vi "Untitled 1.vi"() -> ()   [LabVIEW 2015]
uses:
  Windows/System32/user32.dll
panel:
  out "Binary Netmask":string
  out "String 2":string
  out "Hosts":string
  out "Host max":string
  out "Host min":string
  out "Broadcast":string
  out "Network":string
  out "Wildcard":string
  out "Netmask":string
  out "Address":string
  in  "INFO":T1
  # "."
  # "."
  # "."
  # "(i.e /24)"
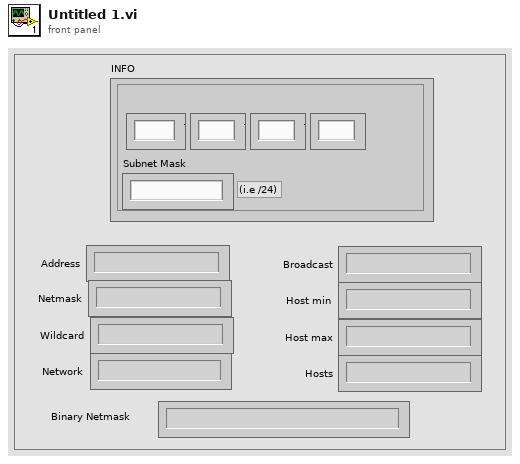
[diagram p1: front panel]
types:
  T1 = cluster{"Subnet Mask":string, "0":string, "1":string, "2":string, "3":string}
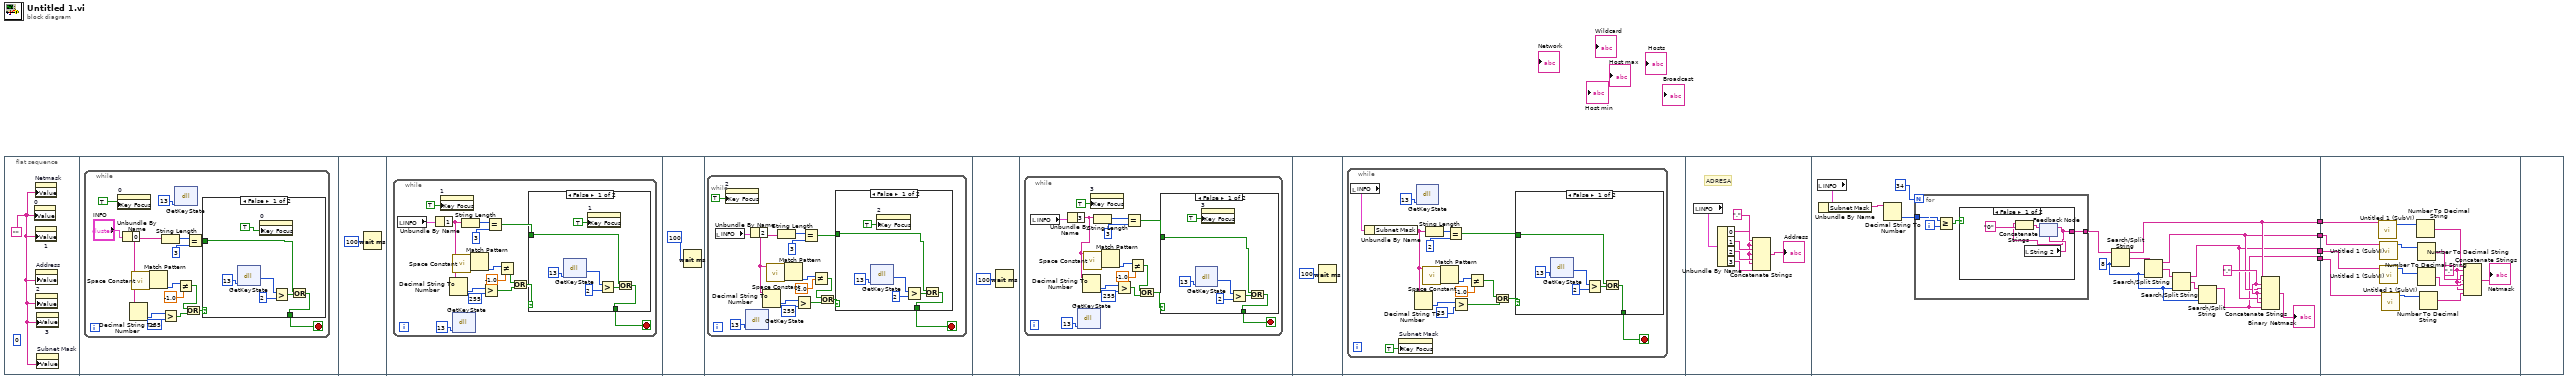
[diagram p0: block diagram]
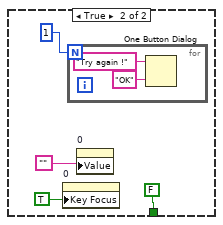
[diagram p2: hidden frame]
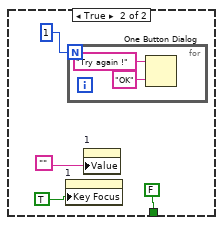
[diagram p3: hidden frame]
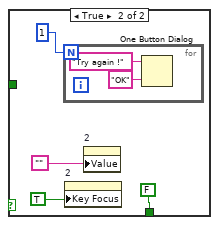
[diagram p4: hidden frame]
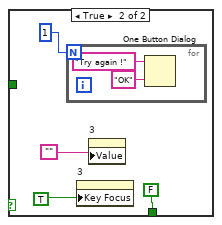
[diagram p5: hidden frame]
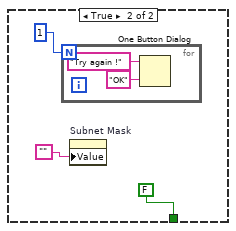
[diagram p6: hidden frame]
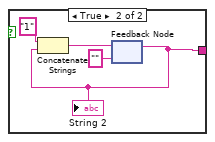
[diagram p7: hidden frame]
diagram:
  n1 = flat-sequence {
    tunnel: [w163] -> w4
    tunnel: [w162] -> w3
    tunnel: [w161] -> w2
    tunnel: [w160] -> w1
    tunnel: w4 -> [w200]
    tunnel: w3 -> [w198]
    tunnel: w2 -> [w197]
    tunnel: w1 -> [w196]
    frame #0 {
      (unwired) 0 ("return type")
      w5 = ""
      n2 = property on="0" class="Str"("Value"=w5) -> ()  [unwired: 2 in, 2 out]
      n3 = property on="Netmask" class="Str"("Value"=w5) -> ()  [unwired: 2 in, 2 out]
      n4 = property on="1" class="Str"("Value"=w5) -> ()  [unwired: 2 in, 2 out]
      n5 = property on="Address" class="Str"("Value"=w5) -> ()  [unwired: 2 in, 2 out]
      n6 = property on="2" class="Str"("Value"=w5) -> ()  [unwired: 2 in, 2 out]
      n7 = property on="3" class="Str"("Value"=w5) -> ()  [unwired: 2 in, 2 out]
      n8 = property on="Subnet Mask" class="Str"("Value"=w5) -> ()  [unwired: 2 in, 2 out]
    }
    frame #1 {
      n9 = while {
        stop <- w15 stop-if-true
        n10 = property on="0" class="Str"("Key Focus"=TRUE) -> ()  [unwired: 2 in, 2 out]
        n11 = Unbundle By Name("INFO") -> ("0"=w11:string)
        n12 = Decimal String To Number(string=w11) -> (number=w17:i32)  [unwired: 2 in, 1 out]
        n13 = call <vilib>:"Space Constant.vi"() -> ("String"=w13:string)
        n14 = Match Pattern(string=w11, regular expression=w13) -> (offset past match=w12:i32)  [unwired: 1 in, 3 out]
        n15 = String Length(string=w11) -> (length=w19:i32)
        n16 = Greater?(x=w17, y=255) -> (0:w9:bool)
        n17 = dll-call lib="C:/Windows/System32/user32.dll" fn="GetKeyState"("vkey"=13) -> ()  [unwired: 5 in, 2 out]
        n18 = Not Equal?(x=w12, y=-1.0) -> (x != y?=w8:bool)
        n19 = Or(x=w8, y=w9) -> (x .or. y?=w7:bool)
        n20 = Equal?(x=w19, y=3) -> (x = y?=w14:bool)
        n21 = case shown="False" w7 {
          tunnel: [w22 FALSE] -> w15
          tunnel: w14 -> [w23 _]
          frame False {
            n22 = dll-call lib="C:/Windows/System32/user32.dll" fn="GetKeyState"("vkey"=13) -> ("return type"=w26:i32)  [unwired: 4 in, 2 out]
            n23 = property on="0" class="Str"("Key Focus"=TRUE) -> ()  [unwired: 2 in, 2 out]
            n24 = Greater?(x=w26, y=2) -> (0:w24:bool)
            n25 = Or(x=w23, y=w24) -> (x .or. y?=w22:bool)
          }
          frame True {
            n26 = property on="0" class="Str"("Key Focus"=TRUE) -> ()  [unwired: 2 in, 2 out]
            n27 = for {
              N: 1 -> [_]
              n28 = One Button Dialog(message="Try again !", button name ("OK")="OK") -> ()  [unwired: 1 out]
            }
            n29 = property on="0" class="Str"("Value"="") -> ()  [unwired: 2 in, 2 out]
          }
        }
      }
    }
    frame #2 {
      n30 = Wait (ms)(milliseconds to wait=u32 100) -> ()  [unwired: 1 out]
    }
    frame #3 {
      n31 = while {
        stop <- w44 stop-if-true
        n32 = local read "INFO"() -> (w51:T1)
        n33 = Unbundle By Name(w51) -> ("1"=w41:string)
        n34 = property on="1" class="Str"("Key Focus"=TRUE) -> ()  [unwired: 2 in, 2 out]
        n35 = Decimal String To Number(string=w41) -> (number=w47:i32)  [unwired: 2 in, 1 out]
        n36 = dll-call lib="C:/Windows/System32/user32.dll" fn="GetKeyState"("vkey"=13) -> ()  [unwired: 5 in, 2 out]
        n37 = call <vilib>:"Space Constant.vi"() -> ("String"=w43:string)
        n38 = String Length(string=w41) -> (length=w50:i32)
        n39 = Match Pattern(string=w41, regular expression=w43) -> (offset past match=w42:i32)  [unwired: 1 in, 3 out]
        n40 = Greater?(x=w47, y=255) -> (0:w39:bool)
        n41 = Equal?(x=w50, y=3) -> (x = y?=w45:bool)
        n42 = Not Equal?(x=w42, y=-1.0) -> (x != y?=w38:bool)
        n43 = Or(x=w38, y=w39) -> (x .or. y?=w40:bool)
        n44 = case shown="False" w40 {
          tunnel: [w52 FALSE] -> w44
          tunnel: w45 -> [w53 _]
          frame False {
            n45 = dll-call lib="C:/Windows/System32/user32.dll" fn="GetKeyState"("vkey"=13) -> ("return type"=w56:i32)  [unwired: 4 in, 2 out]
            n46 = property on="1" class="Str"("Key Focus"=TRUE) -> ()  [unwired: 2 in, 2 out]
            n47 = Greater?(x=w56, y=2) -> (0:w54:bool)
            n48 = Or(x=w53, y=w54) -> (x .or. y?=w52:bool)
          }
          frame True {
            n49 = property on="1" class="Str"("Key Focus"=TRUE) -> ()  [unwired: 2 in, 2 out]
            n50 = for {
              N: 1 -> [_]
              n51 = One Button Dialog(message="Try again !", button name ("OK")="OK") -> ()  [unwired: 1 out]
            }
            n52 = property on="1" class="Str"("Value"="") -> ()  [unwired: 2 in, 2 out]
          }
        }
      }
    }
    frame #4 {
      n53 = Wait (ms)(milliseconds to wait=u32 100) -> ()  [unwired: 1 out]
    }
    frame #5 {
      n54 = while {
        stop <- w74 stop-if-true
        n55 = local read "INFO"() -> (w79:T1)
        n56 = property on="2" class="Str"("Key Focus"=TRUE) -> ()  [unwired: 2 in, 2 out]
        n57 = dll-call lib="C:/Windows/System32/user32.dll" fn="GetKeyState"("vkey"=13) -> ()  [unwired: 5 in, 2 out]
        n58 = Unbundle By Name(w79) -> ("2"=w68:string)
        n59 = Decimal String To Number(string=w68) -> (number=w77:i32)  [unwired: 2 in, 1 out]
        n60 = call <vilib>:"Space Constant.vi"() -> ("String"=w73:string)
        n61 = String Length(string=w68) -> (length=w81:i32)
        n62 = Match Pattern(string=w68, regular expression=w73) -> (offset past match=w72:i32)  [unwired: 1 in, 3 out]
        n63 = Greater?(x=w77, y=255) -> (0:w69:bool)
        n64 = Equal?(x=w81, y=3) -> (x = y?=w75:bool)
        n65 = Not Equal?(x=w72, y=-1.0) -> (x != y?=w70:bool)
        n66 = Or(x=w70, y=w69) -> (x .or. y?=w71:bool)
        n67 = case shown="False" w71 {
          tunnel: [w82 FALSE] -> w74
          tunnel: w75 -> [w83 _]
          frame False {
            n68 = dll-call lib="C:/Windows/System32/user32.dll" fn="GetKeyState"("vkey"=13) -> ("return type"=w86:i32)  [unwired: 4 in, 2 out]
            n69 = property on="2" class="Str"("Key Focus"=TRUE) -> ()  [unwired: 2 in, 2 out]
            n70 = Greater?(x=w86, y=2) -> (0:w84:bool)
            n71 = Or(x=w83, y=w84) -> (x .or. y?=w82:bool)
          }
          frame True {
            n72 = for {
              N: 1 -> [_]
              n73 = One Button Dialog(message="Try again !", button name ("OK")="OK") -> ()  [unwired: 1 out]
            }
            n74 = property on="2" class="Str"("Key Focus"=TRUE) -> ()  [unwired: 2 in, 2 out]
            n75 = property on="2" class="Str"("Value"="") -> ()  [unwired: 2 in, 2 out]
          }
        }
      }
    }
    frame #6 {
      n76 = Wait (ms)(milliseconds to wait=u32 100) -> ()  [unwired: 1 out]
    }
    frame #7 {
      n77 = while {
        stop <- w104 stop-if-true
        n78 = local read "INFO"() -> (w109:T1)
        n79 = Unbundle By Name(w109) -> ("3"=w100:string)
        n80 = dll-call lib="C:/Windows/System32/user32.dll" fn="GetKeyState"("vkey"=13) -> ()  [unwired: 5 in, 2 out]
        n81 = Decimal String To Number(string=w100) -> (number=w107:i32)  [unwired: 2 in, 1 out]
        n82 = call <vilib>:"Space Constant.vi"() -> ("String"=w101:string)
        n83 = property on="3" class="Str"("Key Focus"=TRUE) -> ()  [unwired: 2 in, 2 out]
        n84 = String Length(string=w100) -> (length=w111:i32)
        n85 = Match Pattern(string=w100, regular expression=w101) -> (offset past match=w98:i32)  [unwired: 1 in, 3 out]
        n86 = Greater?(x=w107, y=255) -> (0:w102:bool)
        n87 = Equal?(x=w111, y=3) -> (x = y?=w105:bool)
        n88 = Not Equal?(x=w98, y=-1.0) -> (x != y?=w97:bool)
        n89 = Or(x=w97, y=w102) -> (x .or. y?=w103:bool)
        n90 = case shown="False" w103 {
          tunnel: [w112 FALSE] -> w104
          tunnel: w105 -> [w113 _]
          frame False {
            n91 = dll-call lib="C:/Windows/System32/user32.dll" fn="GetKeyState"("vkey"=13) -> ("return type"=w116:i32)  [unwired: 4 in, 2 out]
            n92 = property on="3" class="Str"("Key Focus"=TRUE) -> ()  [unwired: 2 in, 2 out]
            n93 = Greater?(x=w116, y=2) -> (0:w114:bool)
            n94 = Or(x=w113, y=w114) -> (x .or. y?=w112:bool)
          }
          frame True {
            n95 = for {
              N: 1 -> [_]
              n96 = One Button Dialog(message="Try again !", button name ("OK")="OK") -> ()  [unwired: 1 out]
            }
            n97 = property on="3" class="Str"("Key Focus"=TRUE) -> ()  [unwired: 2 in, 2 out]
            n98 = property on="3" class="Str"("Value"="") -> ()  [unwired: 2 in, 2 out]
          }
        }
      }
    }
    frame #8 {
      n99 = Wait (ms)(milliseconds to wait=u32 100) -> ()  [unwired: 1 out]
    }
    frame #9 {
      n100 = while {
        stop <- w134 stop-if-true
        n101 = local read "INFO"() -> (w141:T1)
        n102 = Unbundle By Name(w141) -> ("Subnet Mask"=w128:string)
        n103 = property on="Subnet Mask" class="Str"("Key Focus"=TRUE) -> ()  [unwired: 2 in, 2 out]
        n104 = Decimal String To Number(string=w128) -> (number=w137:i32)  [unwired: 2 in, 1 out]
        n105 = dll-call lib="C:/Windows/System32/user32.dll" fn="GetKeyState"("vkey"=13) -> ()  [unwired: 5 in, 2 out]
        n106 = call <vilib>:"Space Constant.vi"() -> ("String"=w133:string)
        n107 = String Length(string=w128) -> (length=w140:i32)
        n108 = Match Pattern(string=w128, regular expression=w133) -> (offset past match=w132:i32)  [unwired: 1 in, 3 out]
        n109 = Equal?(x=w140, y=2) -> (x = y?=w135:bool)
        n110 = Greater?(x=w137, y=25) -> (0:w130:bool)
        n111 = Not Equal?(x=w132, y=-1.0) -> (x != y?=w127:bool)
        n112 = Or(x=w127, y=w130) -> (x .or. y?=w129:bool)
        n113 = case shown="False" w129 {
          tunnel: [w142 FALSE] -> w134
          tunnel: w135 -> [w143 _]
          frame False {
            n114 = dll-call lib="C:/Windows/System32/user32.dll" fn="GetKeyState"("vkey"=13) -> ("return type"=w146:i32)  [unwired: 4 in, 2 out]
            n115 = Greater?(x=w146, y=2) -> (0:w144:bool)
            n116 = Or(x=w143, y=w144) -> (x .or. y?=w142:bool)
          }
          frame True {
            n117 = for {
              N: 1 -> [_]
              n118 = One Button Dialog(message="Try again !", button name ("OK")="OK") -> ()  [unwired: 1 out]
            }
            n119 = property on="Subnet Mask" class="Str"("Value"="") -> ()  [unwired: 2 in, 2 out]
          }
        }
      }
    }
    frame #10 {
      w155 = "."
      # "ADRESA"
      n120 = local read "INFO"() -> (w159:T1)
      n121 = Unbundle By Name(w159) -> ("0"=w158:string, "1"=w157:string, "2"=w156:string, "3"=w154:string)
      n122 = Concatenate Strings(w158, w155, w157, w155, w156, w155, w154) -> (→"Address":string)
    }
    frame #11 {
      w165 = "." ("string")
      w166 = 8 ("offset (0)")
      n123 = local read "INFO"() -> (w174:T1)
      n124 = Unbundle By Name(w174) -> ("Subnet Mask"=w173:string)
      n125 = Decimal String To Number(string=w173) -> (number=w171:i32)  [unwired: 2 in, 1 out]
      n126 = for {
        N: 34 -> [_]
        tunnel: [w178] -> w170
        tunnel: w171 -> [w176]
        i -> [w175]
        n127 = Greater Or Equal?(x=w176, y=w175) -> (x >= y?=w177:bool)
        n128 = case shown="False" w177 {
          tunnel: [w179 w183] -> w178
          frame False {
            n129 = local read "String 2"() -> (w180:string)
            n130 = feedback #1(w180) -> (w179:string)
            n131 = Concatenate Strings(w179, "0" ("string")) -> (w181:string)
            n132 = feedback-in #1(w181) -> ()
          }
          frame True {
            n133 = feedback #2("") -> (w183:string)
            "String 2" <- w183
            n134 = Concatenate Strings("1" ("string"), w183) -> (w185:string)
            n135 = feedback-in #2(w185) -> ()
          }
        }
      }
      n136 = Search/Split String(string=w170, offset (0)=w166) -> (substring before match=w163:string, match + rest of string=w169:string)  [unwired: 1 in, 1 out]
      n137 = Search/Split String(string=w169, offset (0)=w166) -> (substring before match=w162:string, match + rest of string=w168:string)  [unwired: 1 in, 1 out]
      n138 = Search/Split String(string=w168, offset (0)=w166) -> (substring before match=w161:string, match + rest of string=w167:string)  [unwired: 1 in, 1 out]
      n139 = Search/Split String(string=w167, offset (0)=w166) -> (substring before match=w160:string)  [unwired: 1 in, 2 out]
      n140 = Concatenate Strings(w163, w165, w162, w165, w161, w165, w160) -> (→"Binary Netmask":string)
    }
    frame #12 {
      w188 = "." ("string")
      n141 = call "Untitled 1 (SubVI).vi"("string"=w200) -> ("number"=w199:u32)  [unwired: 10 in]
      n142 = call "Untitled 1 (SubVI).vi"("string"=w198) -> ("number"=w195:u32)  [unwired: 10 in]
      n143 = call "Untitled 1 (SubVI).vi"("string"=w197) -> ("number"=w194:u32)  [unwired: 10 in]
      n144 = call "Untitled 1 (SubVI).vi"("string"=w196) -> ("number"=w193:u32)  [unwired: 10 in]
      n145 = Number To Decimal String(number=w199) -> (decimal integer string=w191:string)  [unwired: 1 in]
      n146 = Number To Decimal String(number=w195) -> (decimal integer string=w190:string)  [unwired: 1 in]
      n147 = Number To Decimal String(number=w194) -> (decimal integer string=w189:string)  [unwired: 1 in]
      n148 = Number To Decimal String(number=w193) -> (decimal integer string=w187:string)  [unwired: 1 in]
      n149 = Concatenate Strings(w191, w188, w190, w188, w189, w188, w187) -> (→"Netmask":string)
    }
    frame #13 {
    }
  }
